vi "adcOffset_Gain.vi"(2 "CCS Base Folder 2":path=path "C:/ti/ccs1020/ccs/ccs_base", 3 "CCXML File (target configuration)":path=path "D:/Projects/C2000/Grande/c2000_topogrande_avv/bitfield-submodule/common/targetConfigs/TMS320F280039C.ccxml", 4 "program file":path=path "D:/Projects/C2000/Grande/c2000_topogrande_avv/testcases_non_avv/ADC/adc_off-gain/Debug/topog_adc_off-gain.out", 5 "error in (no error)":errorcluster) -> (19 "error out":errorcluster)   [LabVIEW 2019]
uses:
  Ctrls/ADC_LV_Variables.ctl
  Ctrls/ADC_CTRL.ctl
  <userlib>/_TI-LA/Reusable/CCS/APIs/Data/Polymorphics/Write Data To Symbol - U16.vi
  <userlib>/_TI-LA/Reusable/CCS/APIs/CCS.lvlib
  common/Comman_nilesh/File_Write/Data_Logging.lvclass
panel:
  in  "File Directory":path=path "D:/Projects/C2000/Grande/Data/ADC/Offset_Gain"
  in  "ACQPS":u16[](array[numeric])=[8, 38]
  in  "No_Of_Points":i32=5
  in  "Vref_Voltage":dbl=2.5
  in  "ADC_Variables":T1={"ACQPS"=25, "Config_Enable"=1, "Prescale"=2, "ADC"=enum."A", "Adc_Channel"=1, "Ref_Int/EXT"=FALSE}
  out "Pin_Config":i32=2
  out "Programed":bool=TRUE
  in  "Data_File":path=path "D:/Projects/C2000/Grande/Data/ADC/Offset_Gain/New Text Document.txt"
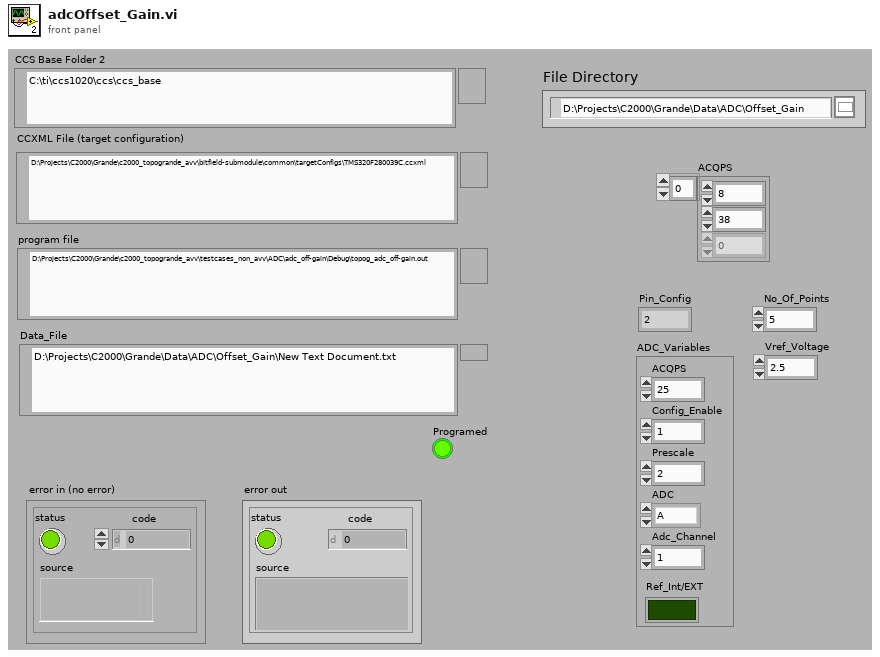
[diagram p1: front panel]
types:
  T1 = typedef "ADC_LV_Variables.ctl" = cluster{"ACQPS":u16, "Config_Enable":u16, "Prescale":u16, "ADC":T2, "Adc_Channel":u16, "Ref_Int/EXT":bool}
  T2 = typedef "ADC_CTRL.ctl" = enum16{"A", "B", "C"}
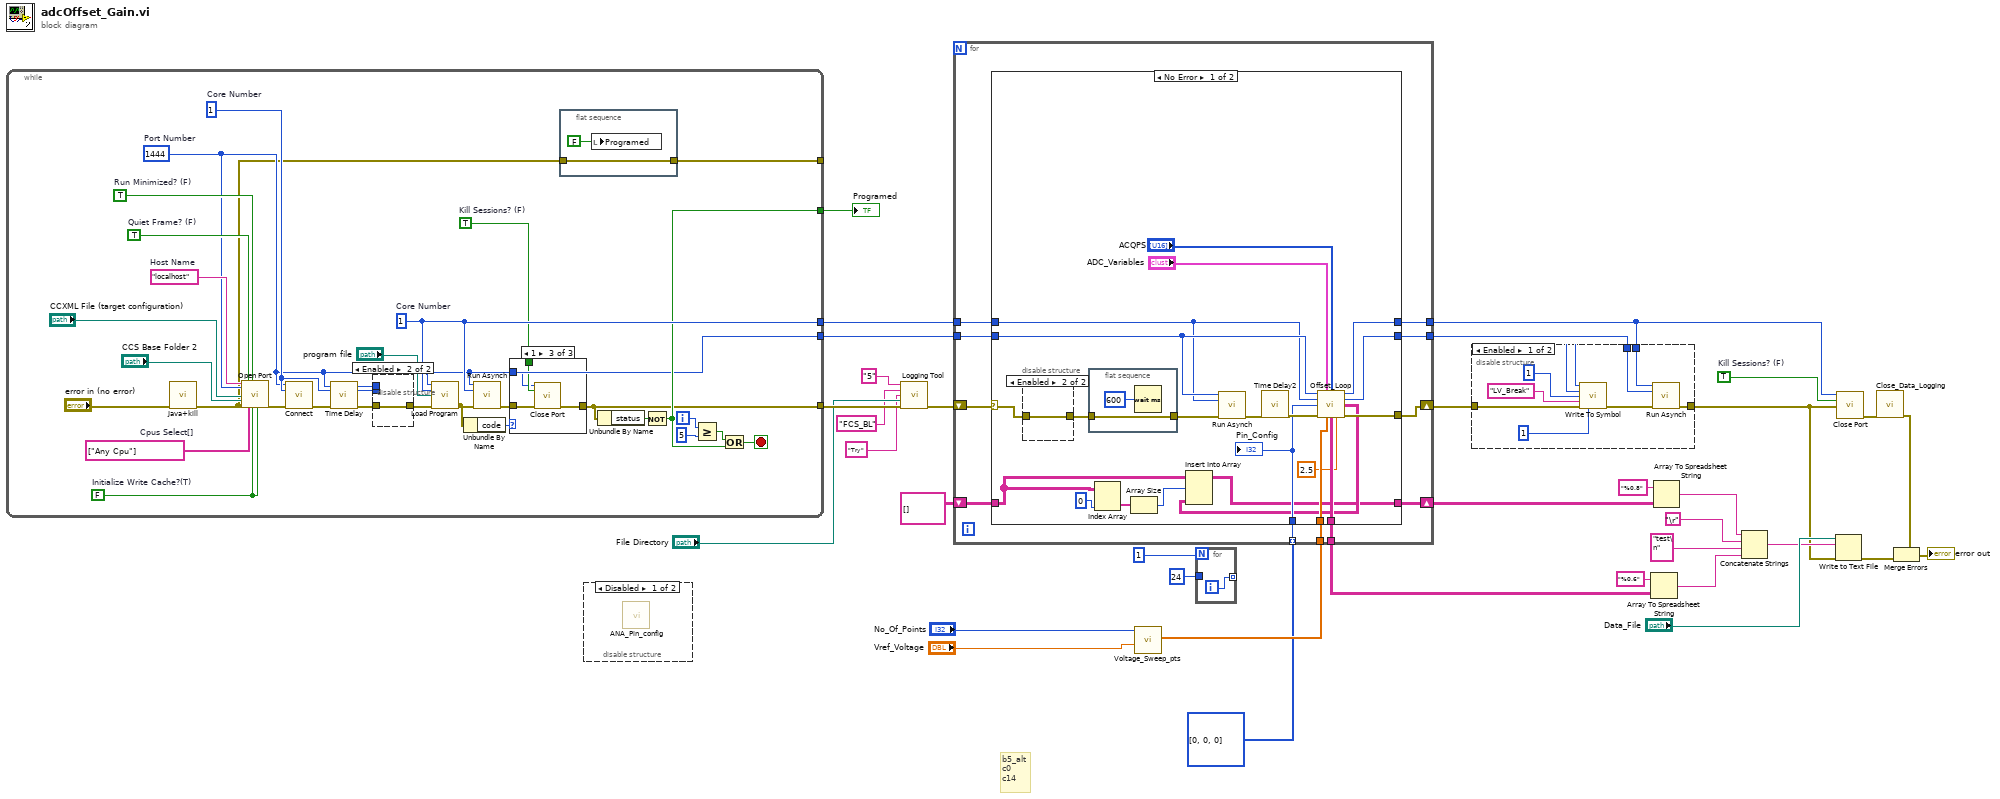
[diagram p0: block diagram]
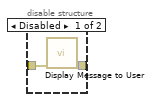
[diagram p4: hidden frame]
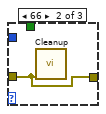
[diagram p7: hidden frame]
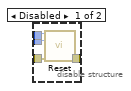
[diagram p8: hidden frame]
diagram:
  w35 = TRUE  # Kill Sessions? (F)
  # "b5_alt\nc0\nc14"
  n1 = while {
    tunnel: [w39] -> w16
    tunnel: [w38] -> w31
    tunnel: [w48] -> w30
    tunnel: [w44] -> w29
    tunnel: [w36] -> _
    i -> [w50]
    stop <- w51 stop-if-true
    w41 = TRUE  # Kill Sessions? (F)
    w48 = u16 1  # Core Number
    w49 = u16 1  # Core Number
    w57 = FALSE  # Initialize Write Cache?(T)
    w58 = string[] ["Any Cpu"]  # Cpus Select[]
    w59 = TRUE  # Run Minimized? (F)
    w60 = TRUE  # Quiet Frame? (F)
    w38 = u16 1444  # Port Number
    w63 = "localhost"  # Host Name
    n2 = call "Java+kill.vi"("error in (no error)"="error in (no error)") -> ("error out"=w37:errorcluster)  [unwired: 10 in]
    n3 = call <userlib>:"Open Port.vi"("Host Name"=w63, "Port Number"=w38, "CCXML File"="CCXML File (target configuration)", "CCS Base Folder"="CCS Base Folder 2", "error in"=w37, "Quiet Frame? (F)"=w60, "Cpus Select[]"=w58, "Run Minimized? (F)"=w59, "Initialize Write Cache?(T)"=w57, "Initialize Symbol Cache?(T)"=w57) -> ("error out"=w64:errorcluster)  [unwired: 7 in, 2 out]
    n4 = call <userlib>:"Connect.vi"("Port Number"=w38, "Core Number"=w49, "error in"=w64) -> ("error out"=w46:errorcluster)  [unwired: 10 in, 2 out]
    n5 = call "Time Delay"("error in (no error)"=w46) -> ("error out"=w45:errorcluster)  [unwired: 10 in]
    n6 = disable-structure shown="Enabled" {
      disable-tunnel: w45 -> [w76 w77]
      disable-tunnel: [w75 w77] -> w56
      disable-tunnel: w49 -> [w74 _]
      disable-tunnel: w38 -> [w73 _]
      frame Disabled {
        n7 = call <userlib>:"Reset.vi"("Port Number"=w73, "Core Number"=w74, "error in"=w76) -> ("error out"=w75:errorcluster)  [unwired: 10 in, 2 out]
      }
      frame Enabled {
      }
    }
    n8 = call <userlib>:"Load Program.vi"("Port Number"=w38, "Core Number"=w48, "Program File Path"="program file", "error in"=w56) -> ("error out"=w43:errorcluster)  [unwired: 7 in, 4 out]
    n9 = Unbundle By Name(w43) -> ("code"=w42:i32)
    n10 = call <userlib>:"Run Asynch.vi"("Port Number"=w38, "Core Number"=w48, "error in"=w43) -> ("error out"=w40:errorcluster)  [unwired: 10 in, 2 out]
    n11 = case shown="1" w42 {
      tunnel: w41 -> [_ _ w72]
      tunnel: w40 -> [w67 w68 w71]
      tunnel: [w67 w68 w70] -> w39
      tunnel: w38 -> [_ _ w69]
      frame Default {
      }
      frame 66 {
        n12 = call <userlib>:"Cleanup.vi"("error in"=w68) -> ()  [unwired: 14 in, 1 out]
      }
      frame 1 {
        n13 = call <userlib>:"Close Port.vi"("Port Number"=w69, "Kill Sessions? (F)"=w72, "error in"=w71) -> ("error out"=w70:errorcluster)  [unwired: 10 in, 2 out]
      }
    }
    n14 = flat-sequence {
      tunnel: w37 -> [w65]
      tunnel: [w65] -> w36
      frame #0 {
        n15 = local write "Programed"(FALSE ("Repeat")) -> ()
      }
    }
    n16 = Unbundle By Name(w39) -> ("status"=w52:bool)
    n17 = Not(x=w52) -> (.not. x?=w44:bool)
    n18 = Greater Or Equal?(x=w50, y=5) -> (x >= y?=w54:bool)
    n19 = Or(x=w54, y=w44) -> (x .or. y?=w51:bool)
  }
  "Programed" <- w29
  n20 = disable-structure shown="Disabled" {
    frame Disabled {
      n21 = call "ANA_Pin_config.vi"() -> ()  [unwired: 8 in, 4 out]
    }
    frame Enabled {
    }
  }
  n22 = call "Logging Tool.vi"("Chip No"="5", "Wafer Split"="FCS_BL" ("Lot Information"), "Run Mode"="Try" ("Lot Information"), "File Directory"="File Directory", "error constant"=w16) -> ("error out"=w15:errorcluster)  [unwired: 6 in, 4 out]
  n23 = call "Voltage_Sweep_pts.vi"("Vref_Voltage"="Vref_Voltage", "Points"="No_Of_Points") -> ("Array"=w25:dbl[])  [unwired: 9 in]
  n24 = for {
    tunnel: w31 -> [w88]
    tunnel: w30 -> [w87]
    tunnel: [w85] -> w6
    tunnel: w25 -> [w84]
    tunnel: [w82] -> w17
    shift-right: [w86] -> w8
    shift-left: w15 -> [w81]
    tunnel: i32[] [0, 0, 0] -> [w80] mode=indexing
    tunnel: [w79] -> w5
    shift-right: [w83] -> w21
    shift-left: string[][] [] ("output array") -> [w78]
    n25 = case shown="No Error" w81 {
      selector: w81 -> [w97 w118]
      tunnel: w88 -> [w102 w116]
      tunnel: w87 -> [w101 w117]
      tunnel: [w109 w118] -> w86
      tunnel: [w107 w117] -> w85
      tunnel: [w106 w116] -> w79
      tunnel: w84 -> [w103 _]
      tunnel: [w90 _] -> w83
      tunnel: [w99 _] -> w82
      tunnel: w80 -> [w96 _]
      tunnel: w78 -> [w95 _]
      frame No Error {
        n26 = disable-structure shown="Enabled" {
          disable-tunnel: [w112 w113] -> w98
          disable-tunnel: w97 -> [w111 w113]
          frame Disabled {
            n27 = call "Display Message to User"("error in (no error)"=w111) -> ("error out"=w112:errorcluster)  [unwired: 9 in, 1 out]
          }
          frame Enabled {
          }
        }
        n28 = flat-sequence {
          tunnel: [w114] -> w110
          tunnel: w98 -> [w114]
          frame #0 {
            n29 = Wait (ms)(milliseconds to wait=u32 600) -> ()  [unwired: 1 out]
          }
        }
        n30 = Index Array(array=w95, index (col)=0 ("index (row)")) -> (element=w93:string[])  [unwired: 1 in]
        n31 = Array Size(array=w93) -> (size(s)=w92:i32)
        n32 = call <userlib>:"Run Asynch.vi"("Port Number"=w102, "Core Number"=w101, "error in"=w110) -> ("error out"=w108:errorcluster)  [unwired: 10 in, 2 out]
        n33 = call "Time Delay2"("error in (no error)"=w108) -> ("error out"=w104:errorcluster)  [unwired: 10 in]
        n34 = call "Offset_Loop.vi"("Port"=w102, "LV_Variables"="ADC_Variables", "ACQPS"="ACQPS", "Core"=w101, "Pin_Config"=w96, "error in"=w104, "Voltage"=w103, "VREF_Measured"=2.5) -> ("Port Number out"=w107:u16, "Core Number out"=w106:u16, "output array"=w91:string[][], "OFF+GAIN"=w99:string[][], "error out"=w109:errorcluster)  [unwired: 3 in]
        n35 = Insert Into Array(array=w95, index (row)=w92, new element=w91) -> (w90:string[][])  [unwired: 1 in]
        "Pin_Config" <- w96
      }
      frame Error {
      }
    }
  }
  n36 = for {
    N: 1 -> [_]
    tunnel: 24 -> [_]
    tunnel: [w119] -> _ mode=indexing
    i -> [w119]
  }
  n37 = disable-structure shown="Enabled" {
    disable-tunnel: w8 -> [w124 w128]
    disable-tunnel: [w122 w128] -> w7
    disable-tunnel: w6 -> [w121 _]
    disable-tunnel: w5 -> [w120 _]
    frame Enabled {
      n38 = call-poly <userlib>:"Write To Symbol.vi"("Port Number"=w121, "Core Number"=w120, "Page"=1, "Symbol Name"="LV_Break", "error in"=w124, "Write Data"=u16 1) -> ("error out"=w123:errorcluster)  [unwired: 7 in, 2 out]
      n39 = call <userlib>:"Run Asynch.vi"("Port Number"=w121, "Core Number"=w120, "error in"=w123) -> ("error out"=w122:errorcluster)  [unwired: 10 in, 2 out]
    }
    frame Disabled {
    }
  }
  n40 = Array To Spreadsheet String(array=w17, 3:"%0.6" ("format string")) -> (spreadsheet string=w26:string)  [unwired: 1 in]
  n41 = Array To Spreadsheet String(array=w21, 3:"%0.8" ("format string")) -> (spreadsheet string=w19:string)  [unwired: 1 in]
  n42 = Concatenate Strings(w19, "\r", "test\n" ("string"), w26) -> (w28:string)
  n43 = Write to Text File(file (use dialog)="Data_File", text=w28, error in=w7) -> (error out=w33:errorcluster)  [unwired: 1 in, 2 out]
  n44 = call <userlib>:"Close Port.vi"("Port Number"=w6, "Kill Sessions? (F)"=w35, "error in"=w7) -> ("error out"=w12:errorcluster)  [unwired: 10 in, 2 out]
  n45 = call "Close_Data_Logging.vi"("error in"=w12) -> ("error out"=w11:errorcluster)  [unwired: 8 in, 2 out]
  n46 = Merge Errors(w11, w33) -> (→"error out":errorcluster)
